vi "Autonomous Independent.vi"() -> ()   [LabVIEW 2014]
doc: "This VI is called when autonomous begins, and will automatically be terminated when autonomous ends. You can carry out timed or sensor driven robot movement independently without needing to return to the caller."
uses:
  <vilib>/Rock Robotics/WPI/Joystick/WPI_JoystickGetSetRefNum.vi
  <vilib>/Rock Robotics/Network Tables/SD Write Numeric Array.vi
  <vilib>/Rock Robotics/WPI/RobotDrive/WPI_RobotDriveGetSetRefNum.vi
  <vilib>/Rock Robotics/WPI/RobotDrive/WPI_RobotDriveMecanumDrive_Cartesian.vi
panel:
  out "Current Movement, for debugging":T1 {"Z Joystick Value" scale=-1.0..1.0; "Y Joystick Value" scale=1.0..-1.0; "X Joystick Value" scale=-1.0..1.0}
  in  "Array of robot movements":T2(array[cluster]) {"Z Joystick Value" scale=-1.0..1.0; "Y Joystick Value" scale=1.0..-1.0; "X Joystick Value" scale=-1.0..1.0}
  # "Be sure to right-click and choose Data Operations>>Make Current Value default if you want to save the array values with the VI"
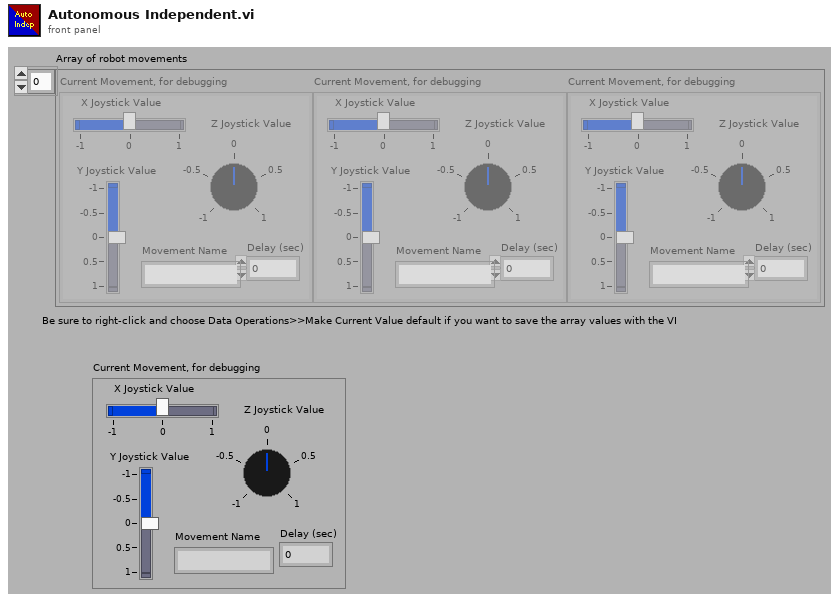
[diagram p1: front panel]
types:
  T1 = cluster{"X Joystick Value":dbl, "Y Joystick Value":dbl, "Z Joystick Value":dbl, "Delay (sec)":dbl, "Movement Name":string}
  T2 = cluster{"X Joystick Value":dbl, "Y Joystick Value":dbl, "Z Joystick Value":dbl, "Delay (sec)":dbl, "Movement Name":string}[]
  T3 = typedef "WPI_JoystickDevRef.ctl" = cluster{"Device":T4}
  T4 = typedef "WPI_JoystickDeviceEnum.ctl" = enum16{"USB 0", "USB 1", "USB 2", "USB 3", "USB 4", "USB 5"}
  T5 = typedef "WPI_RobotDriveDevRef.ctl" = cluster{"DevStatus":errorcluster, "Motors[]":T6[], "Square Inputs":bool, "Max Output":dbl}
  T6 = typedef "WPI_MotorControlDeviceRef.ctl" = cluster{"DeviceStatus":errorcluster, "Type":T7, "PWM":cluster{"Controller":T8, "PWM Channel":T9, "DeadBand":T10}, "CAN":cluster{"Device Number":u8, "Control Mode":T11, "Semaphore":T12, "Max Vout":dbl, "TalonSRX Control Mode":T13}, "Invert":bool, "TransformRef":T14, "InvTransformRef":T14}
  T7 = typedef "WPI_MotorControlType.ctl" = enum16{"PWM", "CAN", "CANTalonSRX"}
  T8 = typedef "FPGA_TypedefDigitalModule.ctl" = enum16{"Controller 1"}
  T9 = typedef "FPGA_DIOPWMChannel.ctl" = enum8{"PWM 0", "PWM 1", "PWM 2", "PWM 3", "PWM 4", "PWM 5", "PWM 6", "PWM 7", "PWM 8", "PWM 9", "PWM MXP 0", "PWM MXP 1", "PWM MXP 2", "PWM MXP 3", "PWM MXP 4", "PWM MXP 5", "PWM MXP 6", "PWM MXP 7", "PWM MXP 8", "PWM MXP 9", "Invalid"}
  T10 = typedef "WPI_PWMDeadband.ctl" = cluster{"Name":string, "maxPositivePwm":i32, "minPositivePwm":i32, "centerPwm":i32, "maxNegativePwm":i32, "minNegativePwm":i32, "angularRange":u16}
  T11 = typedef "WPI_CANJaguar_ControlMode.ctl" = enum8{"Percent VBus", "Current", "Speed", "Position", "Voltage"}
  T12 = typedef "Semaphore RefNum" = refnum<k1>
  T13 = typedef "WPI_CANTalonSRX_APIControlMode.ctl" = enum8{"Percent VBus", "Speed", "Position", "Slave", "Unchanged / Invalid"}
  T14 = typedef "WPI_PWMTransform_ConPane.ctl" = refnum<vi>
  T15 = typedef "WPI_DigitalInputDevRef.ctl" = cluster{"DevStatus":errorcluster, "DIO Channel":T16, "Controller":T8}
  T16 = typedef "FPGA_DIOChannel.ctl" = enum8{"DIO 0", "DIO 1", "DIO 2", "DIO 3", "DIO 4", "DIO 5", "DIO 6", "DIO 7", "DIO 8", "DIO 9", "DIO MXP 0", "DIO MXP 1", "DIO MXP 2", "DIO MXP 3", "DIO MXP 4", "DIO MXP 5", "DIO MXP 6", "DIO MXP 7", "DIO MXP 8", "DIO MXP 9", "DIO MXP 10", "DIO MXP 11", "DIO MXP 12", "DIO MXP 13", "DIO MXP 14", "DIO MXP 15", "Invalid"}
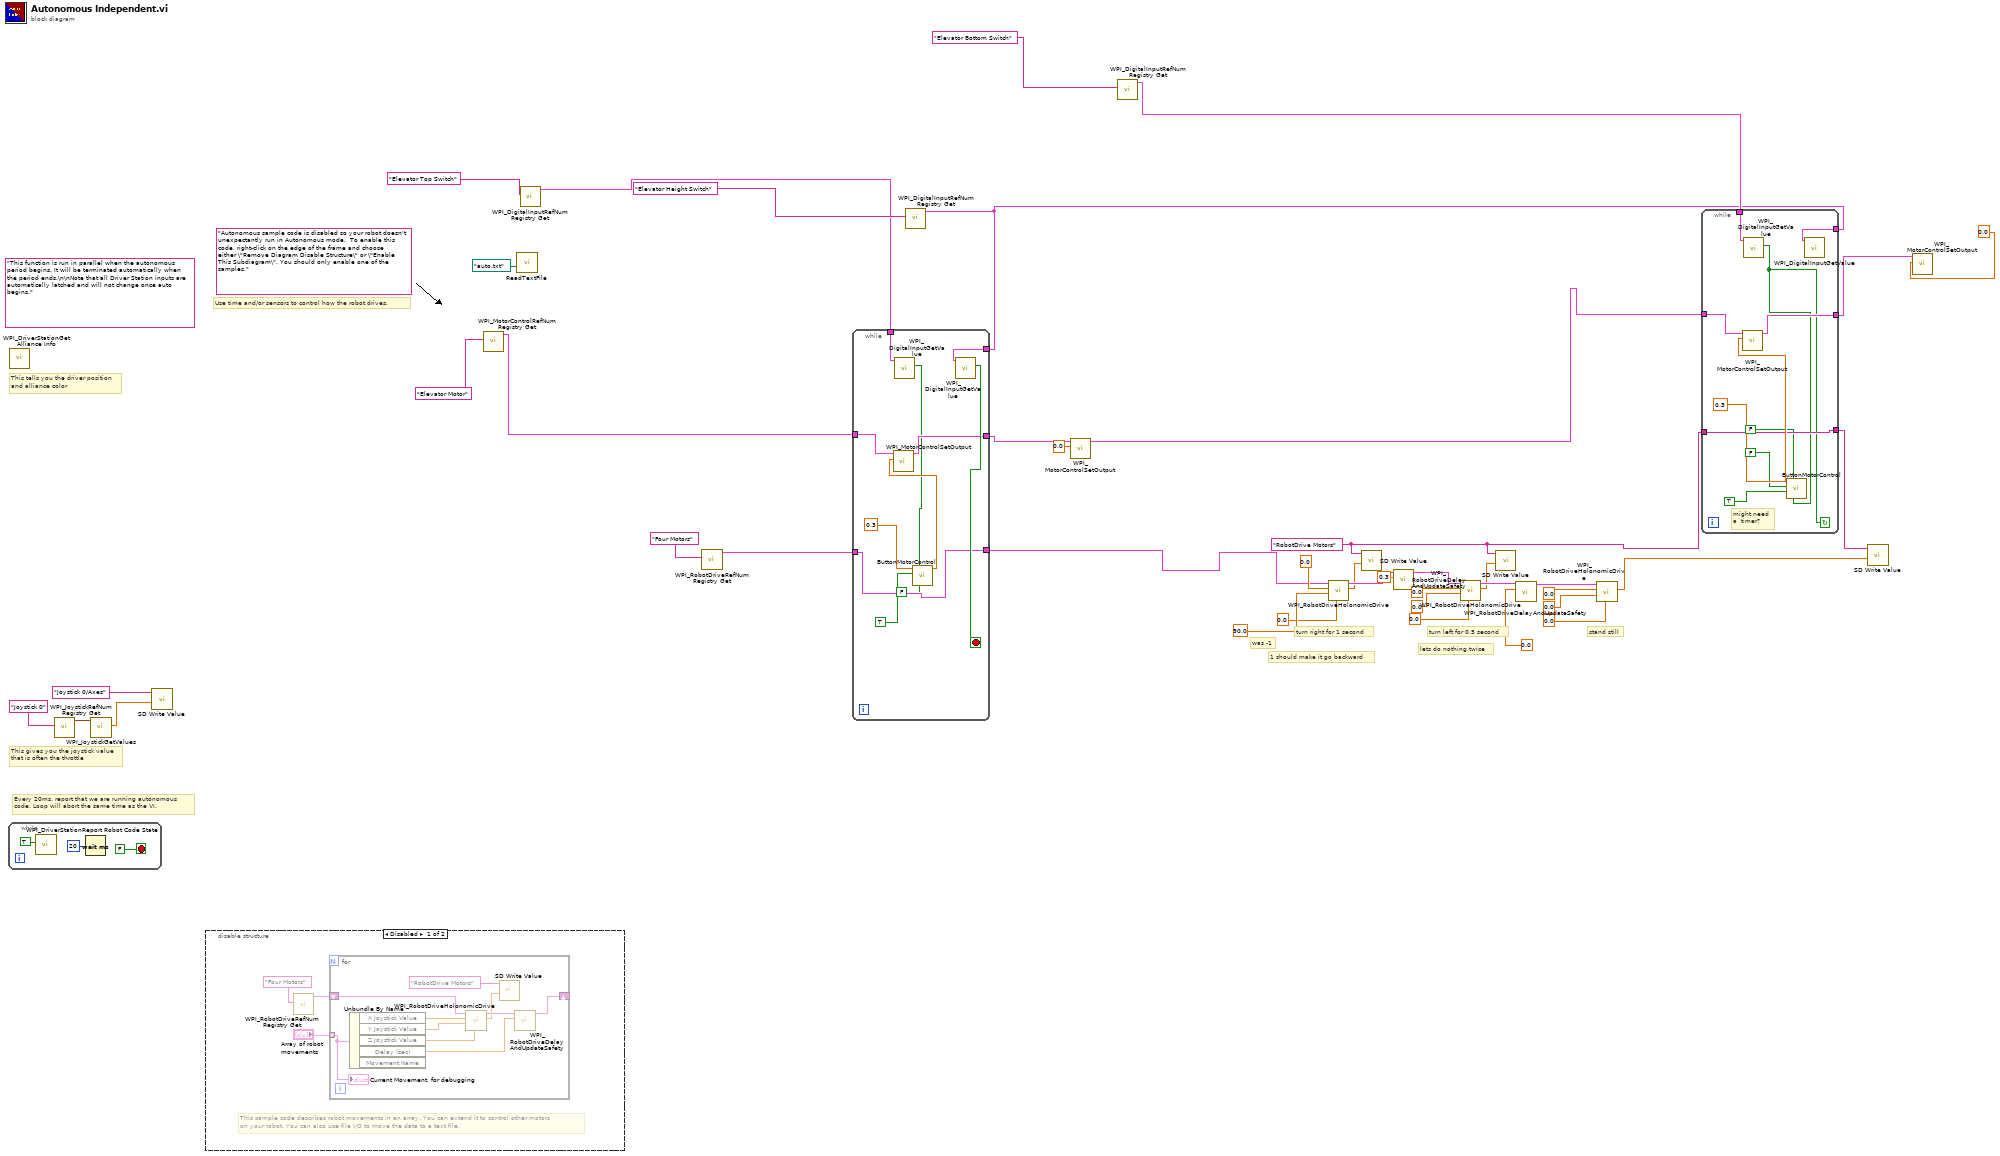
[diagram p0: block diagram]
diagram:
  w4 = "RobotDrive Motors" ("Name")
  (unwired) "Autonomous sample code is disabled so your robot doesn't unexpectantly run in Autonomous mode.  To enable this code, right-click on the edge of the frame and choose either \"Remove Diagram Disable Structure\" or \"Enable This Subdiagram\". You should only enable one of the samples."
  (unwired) "This function is run in parallel when the autonomous period begins. It will be terminated automatically when the period ends.\n\nNote that all Driver Station inputs are automatically latched and will not change once auto begins."
  # "lets do nothing twice"
  # "1 should make it go backward"
  # "was -1"
  # "stand still"
  # "turn left for 0.5 second"
  # "turn right for 1 second"
  # "Every 20ms, report that we are running autonomous\ncode. Loop will abort the same time as the VI."
  # "This gives you the joystick value\nthat is often the throttle"
  # "Use time and/or sensors to control how the robot drives."
  # "This tells you the driver position\nand alliance color"
  n1 = while {
    stop <- FALSE stop-if-true
    n2 = call <vilib>:"WPI_DriverStationReport Robot Code State.vi"("Autonomous"=TRUE) -> ()  [unwired: 10 in, 1 out]
    n3 = Wait (ms)(milliseconds to wait=u32 20) -> ()  [unwired: 1 out]
  }
  n4 = call <vilib>:"WPI_DriverStationGet Alliance Info.vi"() -> ()  [unwired: 12 out]
  n5 = call <vilib>:"WPI_JoystickRefNum Registry Get.vi"("refnum name"="Joystick 0") -> ("JoystickDevRef"=w40:T3)  [unwired: 1 in, 9 out]
  n6 = call <vilib>:"WPI_JoystickGetValues.vi"("JoystickDevRef"=w40) -> ("Axes"=w38:dbl[])  [unwired: 6 in, 4 out]
  n7 = call-poly <vilib>:"SD Write Value.vi"("Numeric Array"=w38, "Name"="Joystick 0/Axes") -> ()  [unwired: 8 in, 2 out]
  n8 = disable-structure shown="Disabled" {
    frame Disabled {
      # "This sample code describes robot movements in an array. You can extend it to control other motors\non your robot. You can also use file I/O to move the data to a text file."
      n9 = call <vilib>:"WPI_RobotDriveRefNum Registry Get.vi"("refnum name"="Four Motors") -> ("RobotDriveDevRef"=w46:T5)  [unwired: 1 in, 9 out]
      n10 = for {
        shift-right: [w54] -> _
        shift-left: w46 -> [w55]
        tunnel: "Array of robot movements" -> [w50] mode=indexing
        n11 = Unbundle By Name(w50) -> ("X Joystick Value"=w53:dbl, "Y Joystick Value"=w52:dbl, "Z Joystick Value"=w49:dbl, "Delay (sec)"=w51:dbl)  [unwired: 1 out]
        n12 = call-poly <vilib>:"WPI_RobotDriveHolonomicDrive.vi"("Rotation"=w49, "Y"=w52, "X"=w53, "RobotDriveDevRef"=w55) -> ("Motor Values"=w48:dbl[], "RobotDriveDevRef"=w56:T5)  [unwired: 5 in, 1 out]
        n13 = call-poly <vilib>:"SD Write Value.vi"("Numeric Array"=w48, "Name"="RobotDrive Motors") -> ()  [unwired: 8 in, 2 out]
        n14 = call <vilib>:"WPI_RobotDriveDelayAndUpdateSafety.vi"("Delay (s)"=w51, "RobotDriveDevRef"=w56) -> ("RobotDriveDevRef 2"=w54:T5)  [unwired: 8 in, 1 out]
        "Current Movement, for debugging" <- w50
      }
    }
    frame Enabled {
    }
  }
  n15 = call <vilib>:"WPI_MotorControlRefNum Registry Get.vi"("refnum name"="Elevator Motor") -> ("MotorControlDevRef"=w14:T6)  [unwired: 9 in, 1 out]
  n16 = call "ReadTextFile.vi"("file (use dialog)"=path "/auto.txt") -> ()  [unwired: 9 in, 2 out]
  n17 = call <vilib>:"WPI_DigitalInputRefNum Registry Get.vi"("refnum name"="Elevator Top Switch") -> ("DigitalInputDevRef"=w15:T15)  [unwired: 9 in, 1 out]
  n18 = call <vilib>:"WPI_RobotDriveRefNum Registry Get.vi"("refnum name"="Four Motors") -> ("RobotDriveDevRef"=w11:T5)  [unwired: 1 in, 9 out]
  n19 = call <vilib>:"WPI_DigitalInputRefNum Registry Get.vi"("refnum name"="Elevator Height Switch") -> ("DigitalInputDevRef"=w2:T15)  [unwired: 9 in, 1 out]
  n20 = while {
    tunnel: w2 -> [w68]
    tunnel: w15 -> [w66]
    tunnel: w14 -> [w65]
    tunnel: [w61] -> w13
    tunnel: [w60] -> w10
    tunnel: w11 -> [w60]
    stop <- w67 stop-if-true
    n21 = call <vilib>:"WPI_DigitalInputGetValue.vi"("DigitalInputDevRef"=w66) -> ("Value"=w59:bool)  [unwired: 8 in, 2 out]
    n22 = call "ButtonMotorControl.vi"("Allow Down"=FALSE, "Allow Up"=w59, "Up"=TRUE, "Speed"=0.3 ("Motor Speed")) -> ("Motor Speed"=w62:dbl)  [unwired: 7 in]
    n23 = call <vilib>:"WPI_MotorControlSetOutput.vi"("Output"=w62, "MotorControlDevRef"=w65) -> ("MotorControlDevRef"=w61:T6)  [unwired: 7 in, 2 out]
    n24 = call <vilib>:"WPI_DigitalInputGetValue.vi"("DigitalInputDevRef"=w68) -> ("Value"=w67:bool)  [unwired: 8 in, 2 out]
  }
  n25 = call <vilib>:"WPI_MotorControlSetOutput.vi"("Output"=0.0, "MotorControlDevRef"=w13) -> ("MotorControlDevRef"=w1:T6)  [unwired: 7 in, 2 out]
  n26 = call <vilib>:"WPI_DigitalInputRefNum Registry Get.vi"("refnum name"="Elevator Bottom Switch") -> ("DigitalInputDevRef"=w8:T15)  [unwired: 9 in, 1 out]
  n27 = call-poly <vilib>:"WPI_RobotDriveHolonomicDrive.vi"("Rotation"=0.0, "Y"=90.0 ("X axis value"), "X"=0.0 ("X axis value"), "RobotDriveDevRef"=w10) -> ("Motor Values"=w22:dbl[], "RobotDriveDevRef"=w31:T5)  [unwired: 5 in, 1 out]
  n28 = call-poly <vilib>:"SD Write Value.vi"("Numeric Array"=w22, "Name"=w4) -> ()  [unwired: 8 in, 2 out]
  n29 = call <vilib>:"WPI_RobotDriveDelayAndUpdateSafety.vi"("Delay (s)"=0.3, "RobotDriveDevRef"=w31) -> ("RobotDriveDevRef 2"=w30:T5)  [unwired: 8 in, 1 out]
  n30 = call-poly <vilib>:"WPI_RobotDriveHolonomicDrive.vi"("Rotation"=0.0, "Y"=0.0 ("X axis value"), "X"=0.0 ("X axis value"), "RobotDriveDevRef"=w30) -> ("Motor Values"=w21:dbl[], "RobotDriveDevRef"=w29:T5)  [unwired: 5 in, 1 out]
  n31 = call-poly <vilib>:"SD Write Value.vi"("Numeric Array"=w21, "Name"=w4) -> ()  [unwired: 8 in, 2 out]
  n32 = call <vilib>:"WPI_RobotDriveDelayAndUpdateSafety.vi"("Delay (s)"=0.0, "RobotDriveDevRef"=w29) -> ("RobotDriveDevRef 2"=w28:T5)  [unwired: 8 in, 1 out]
  n33 = call-poly <vilib>:"WPI_RobotDriveHolonomicDrive.vi"("Rotation"=0.0 ("X axis value"), "Y"=0.0 ("X axis value"), "X"=0.0 ("X axis value"), "RobotDriveDevRef"=w28) -> ("Motor Values"=w20:dbl[])  [unwired: 5 in, 2 out]
  n34 = while {
    tunnel: w2 -> [w79]
    tunnel: w8 -> [w78]
    tunnel: w1 -> [w77]
    tunnel: [w74] -> w5
    tunnel: [w73] -> w3
    tunnel: w4 -> [w73]
    stop <- w69 continue-if-true
    # "might need\na  timer?"
    n35 = call <vilib>:"WPI_DigitalInputGetValue.vi"("DigitalInputDevRef"=w78) -> ("Value"=w69:bool)  [unwired: 8 in, 2 out]
    n36 = call "ButtonMotorControl.vi"("Allow Down"=w69, "Allow Up"=FALSE, "Down"=TRUE ("Up"), "Up"=FALSE, "Speed"=0.3 ("Motor Speed")) -> ("Motor Speed"=w75:dbl)  [unwired: 6 in]
    n37 = call <vilib>:"WPI_MotorControlSetOutput.vi"("Output"=w75, "MotorControlDevRef"=w77) -> ("MotorControlDevRef"=w74:T6)  [unwired: 7 in, 2 out]
    n38 = call <vilib>:"WPI_DigitalInputGetValue.vi"("DigitalInputDevRef"=w79) -> ()  [unwired: 8 in, 3 out]
  }
  n39 = call-poly <vilib>:"SD Write Value.vi"("Numeric Array"=w20, "Name"=w3) -> ()  [unwired: 8 in, 2 out]
  n40 = call <vilib>:"WPI_MotorControlSetOutput.vi"("Output"=0.0, "MotorControlDevRef"=w5) -> ()  [unwired: 7 in, 3 out]
